vi "direction.vi"(2 "?":T1(radio), 3 "speed":i32(knob) scale=0.0..5.0, 4 "Y":dbl, 5 "X":dbl) -> (0 "yResult":dbl, 1 "xResult":dbl)   [LabVIEW 2013]
panel:
  in  "angle":i32
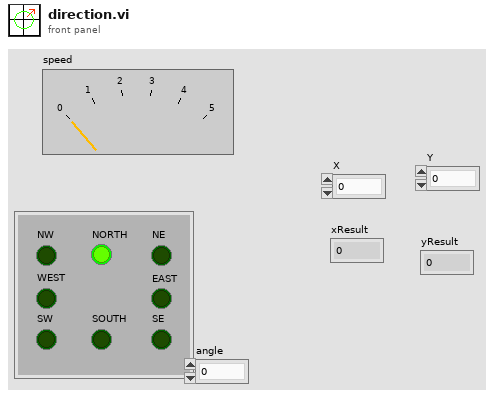
[diagram p1: front panel]
types:
  T1 = enum32{"NORTH", "NE ", "NW", "WEST", "SE", "EAST", "SW", "SOUTH"}
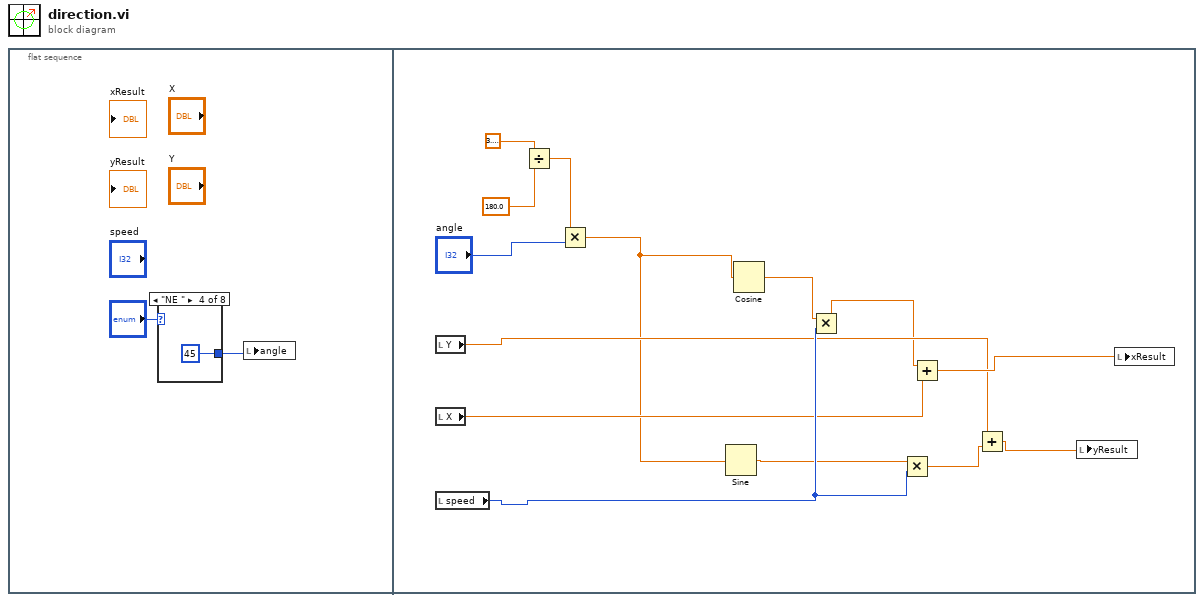
[diagram p0: block diagram]
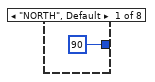
[diagram p2: hidden frame]
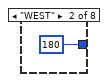
[diagram p3: hidden frame]
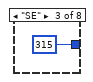
[diagram p4: hidden frame]
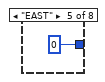
[diagram p5: hidden frame]
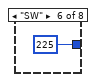
[diagram p6: hidden frame]
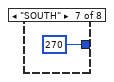
[diagram p7: hidden frame]
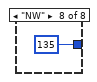
[diagram p8: hidden frame]
diagram:
  n1 = flat-sequence {
    frame #0 {
      n2 = case shown="\"NE \"" "?" {
        tunnel: [90 180 315 45 0 225 270 135] -> w1
        frame "NORTH", Default {
        }
        frame "WEST" {
        }
        frame "SE" {
        }
        frame "NE " {
        }
        frame "EAST" {
        }
        frame "SW" {
        }
        frame "SOUTH" {
        }
        frame "NW" {
        }
      }
      n3 = local write "angle"(w1) -> ()
    }
    frame #1 {
      n4 = local read "Y"() -> (w20:dbl)
      n5 = local read "X"() -> (w21:dbl)
      n6 = local read "speed"() -> (w22:i32)
      n7 = Divide(x=3.141592653589793, y=180.0) -> (x/y=w15:dbl)
      n8 = Multiply(x=w15, y="angle") -> (x*y=w16:dbl)
      n9 = Sine(x=w16) -> (sin(x)=w18:dbl)
      n10 = Cosine(x=w16) -> (cos(x)=w17:dbl)
      n11 = Multiply(x=w17, y=w22) -> (x*y=w11:dbl)
      n12 = Multiply(x=w18, y=w22) -> (x*y=w12:dbl)
      n13 = Add(x=w11, y=w21) -> (x+y=w23:dbl)
      n14 = Add(x=w20, y=w12) -> (x+y=w24:dbl)
      n15 = local write "yResult"(w24) -> ()
      n16 = local write "xResult"(w23) -> ()
    }
  }
